vi "Login_Process.vi"(8 "error in (no error)":errorcluster, 11 "TopLevel in":refnum<class "TopLevel.lvclass">) -> (0 "error out":errorcluster, 3 "TopLevel out":refnum<class "TopLevel.lvclass">)   [LabVIEW 2022 SP3, in "TopLevel.lvclass"]
uses:
  TopLevel.lvclass
  Typedefs/UserLevel_withoutNone--Enum.ctl
  Typedefs/UserLevel--Enum.ctl
panel:
  out "Status":string
  in  "UserLevel":T1
  in  "LogIN":bool
  in  "Cancel":bool
  in  "Password":string
  in  "OK":bool
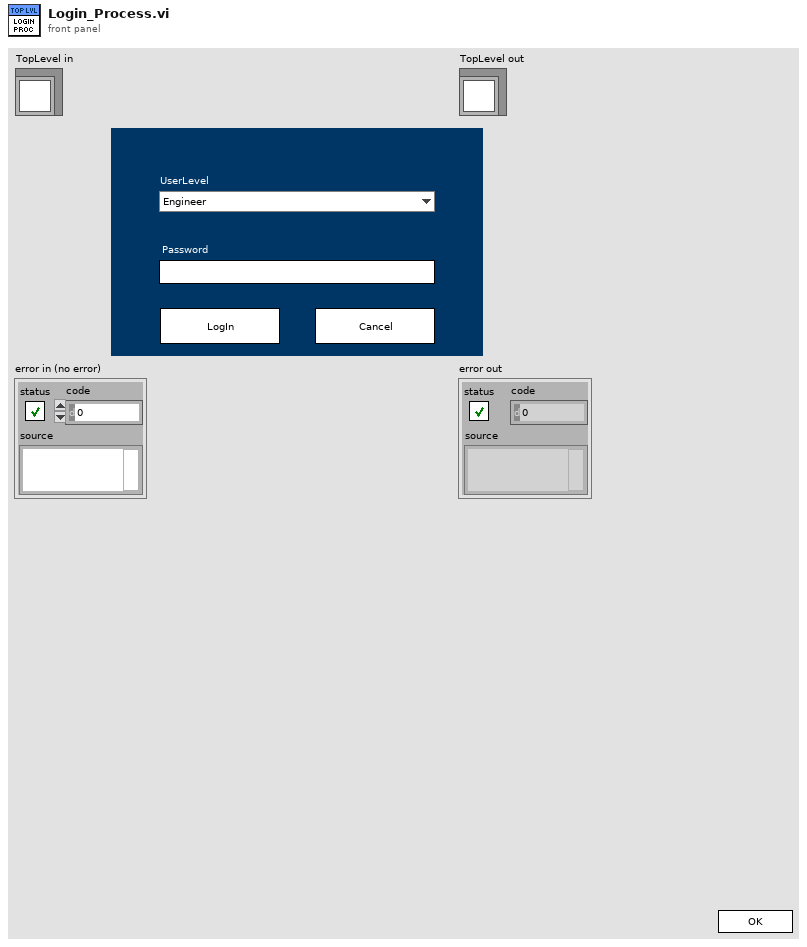
[diagram p1: front panel]
types:
  T1 = typedef "UserLevel_withoutNone--Enum.ctl" = enum16{"Engineer"}
  T2 = typedef "UserLevel--Enum.ctl" = enum16{"None", "Operator", "Engineer"}
  T3 = enum32{"Invalid", "Standard", "Closed", "Hidden", "Minimized", "Maximized"}
  T4 = enum32{"invalid app kind", "Development System", "Run Time System", "Student Edition", "Embedded LabVIEW", "Evaluation", "Custom"}
  T5 = cluster{"Core":cluster{"Current VI Reference":refnum<vi>, "Close Panel on Exit?":bool}, "TopLevel in":refnum<class "TopLevel.lvclass">, "Your string data":string}
  T6 = cluster{"Current VI Reference":refnum<vi>, "Close Panel on Exit?":bool}
  T7 = typedef "TopLevel.lvclass/UserEvents.ctl" = cluster{"API Incoming Event":refnum<user-event>, "API Executed Event":refnum<user-event>, "API Return Event":refnum<user-event>, "Exit Event":refnum<user-event>, "StatusChanged":refnum<user-event>, "DLP GUI Config Changed":refnum<user-event>, "AppEvent":refnum<user-event>, "Login Event":refnum<user-event>, "HeadPrimeStatusEvent":refnum<user-event>}
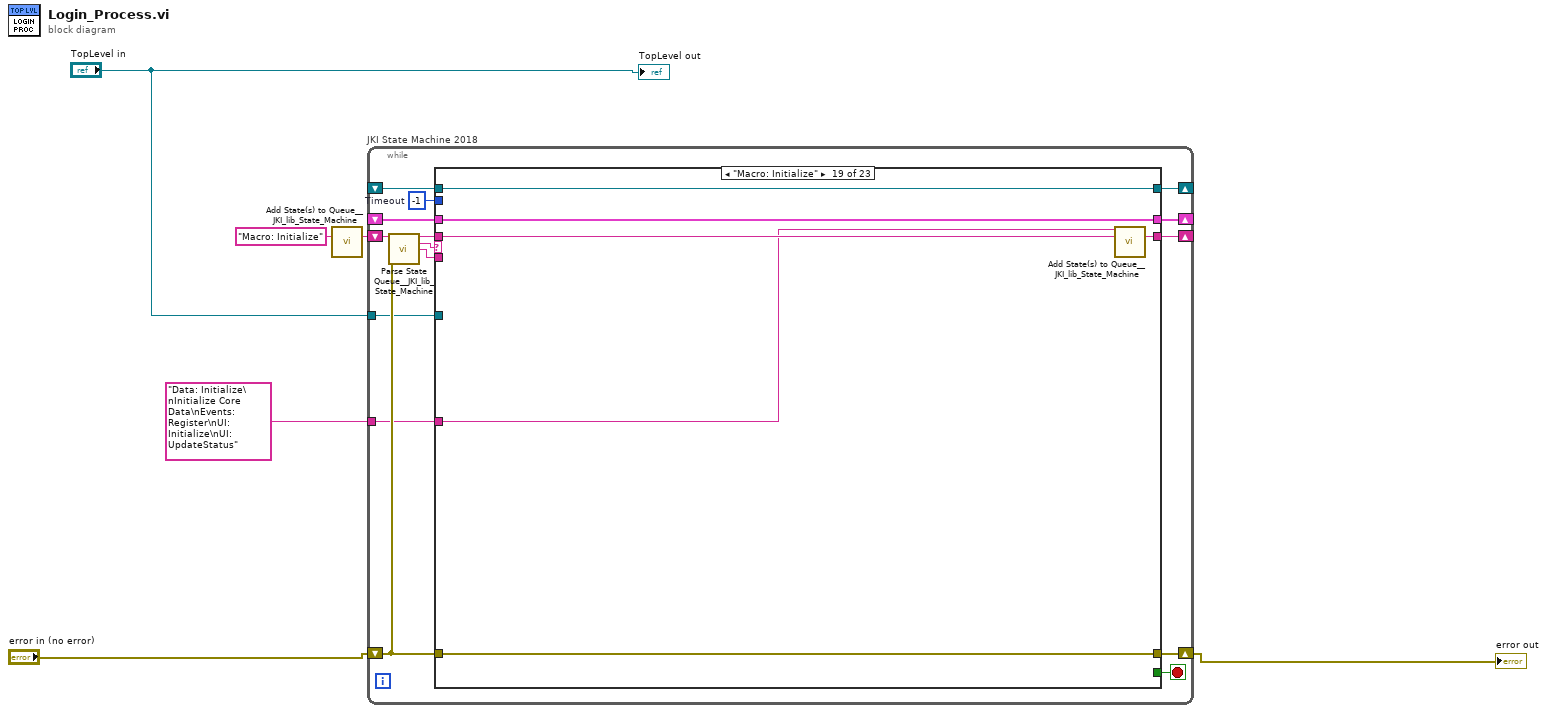
[diagram p0: block diagram]
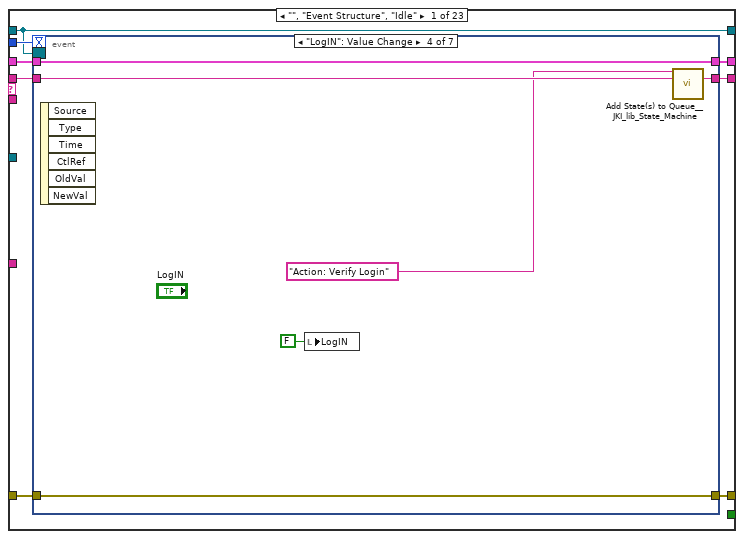
[diagram p2: hidden frame]
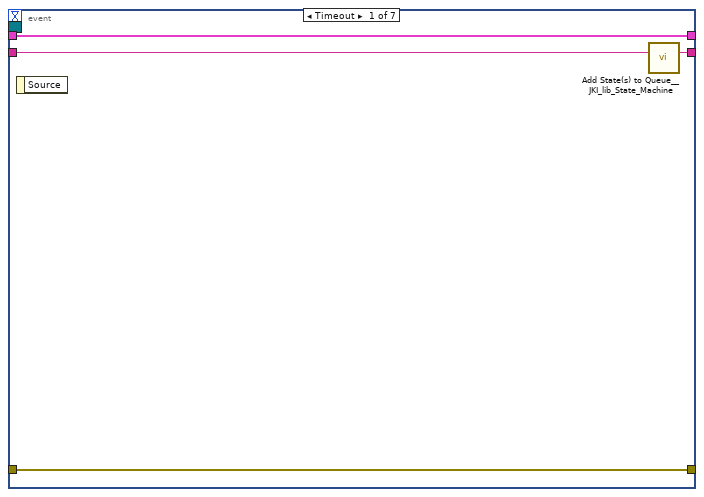
[diagram p3: hidden frame]
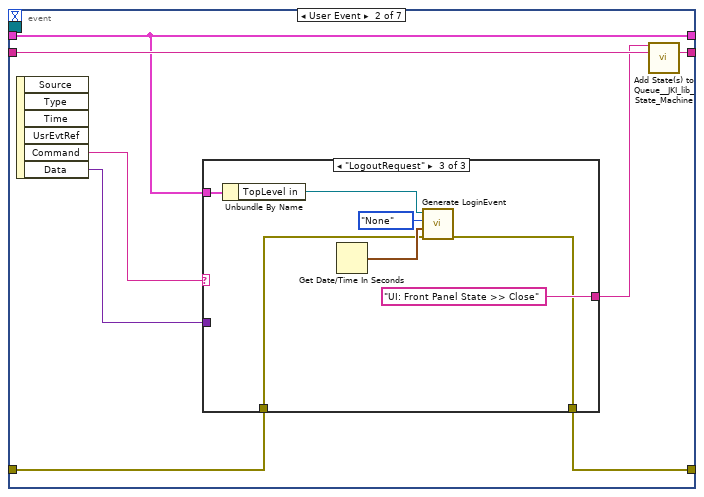
[diagram p4: hidden frame]
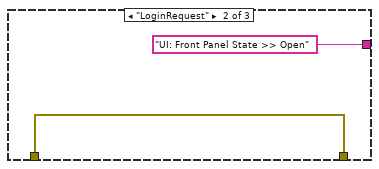
[diagram p6: hidden frame]
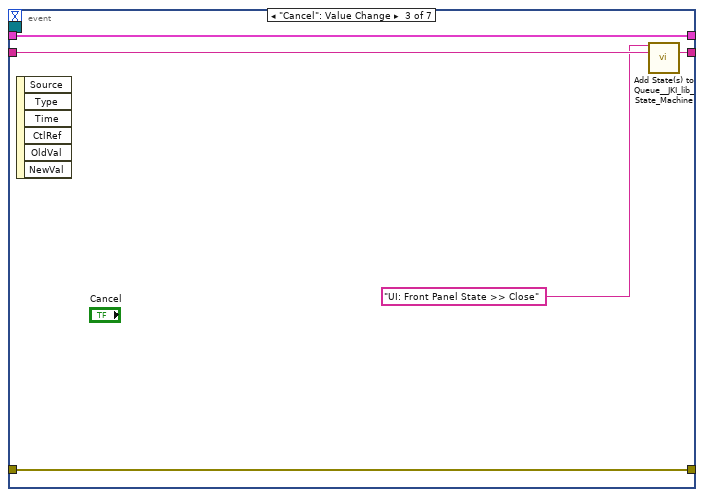
[diagram p7: hidden frame]
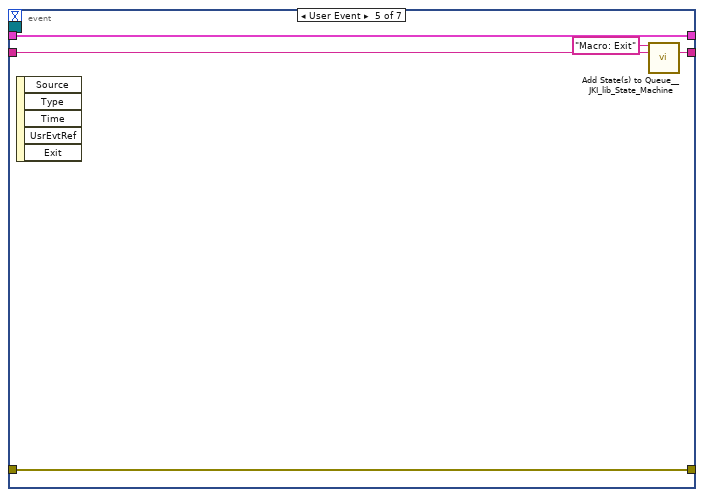
[diagram p8: hidden frame]
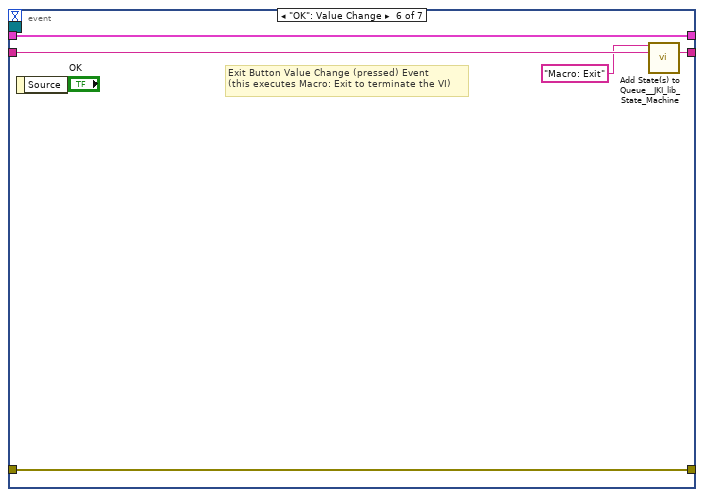
[diagram p9: hidden frame]
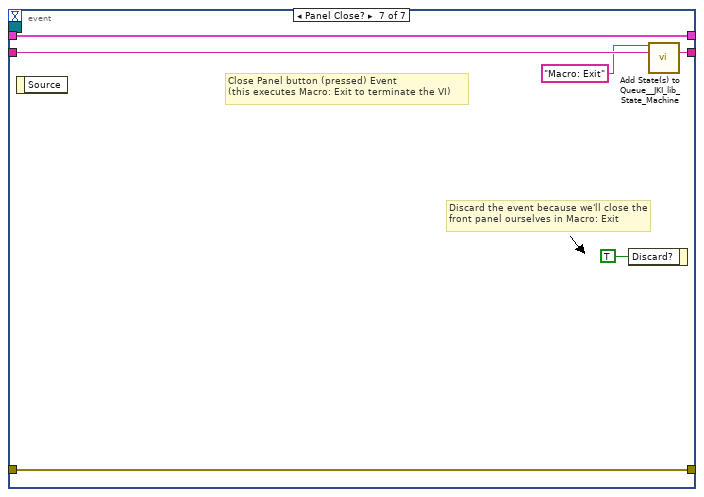
[diagram p10: hidden frame]
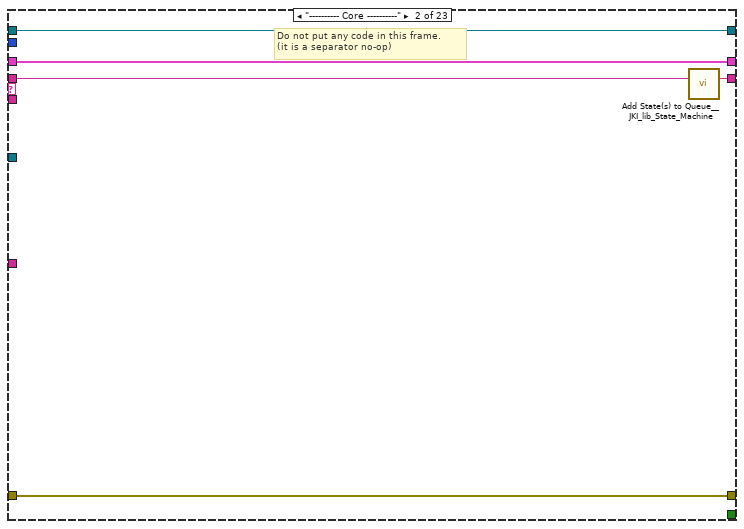
[diagram p11: hidden frame]
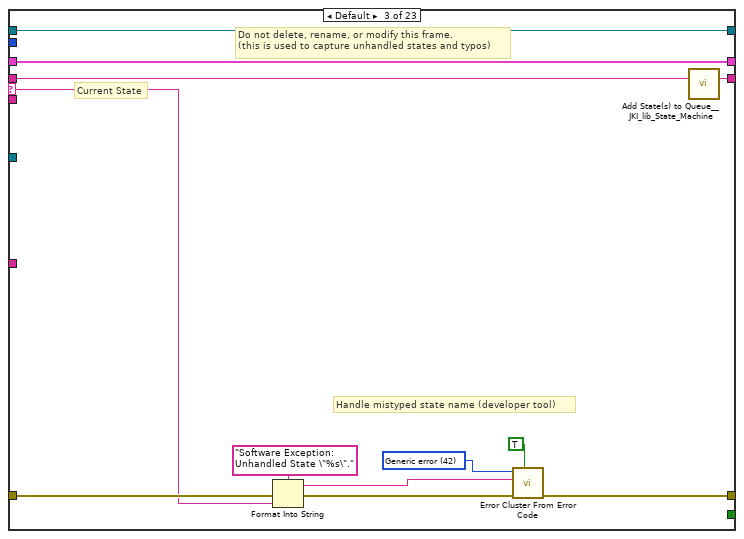
[diagram p12: hidden frame]
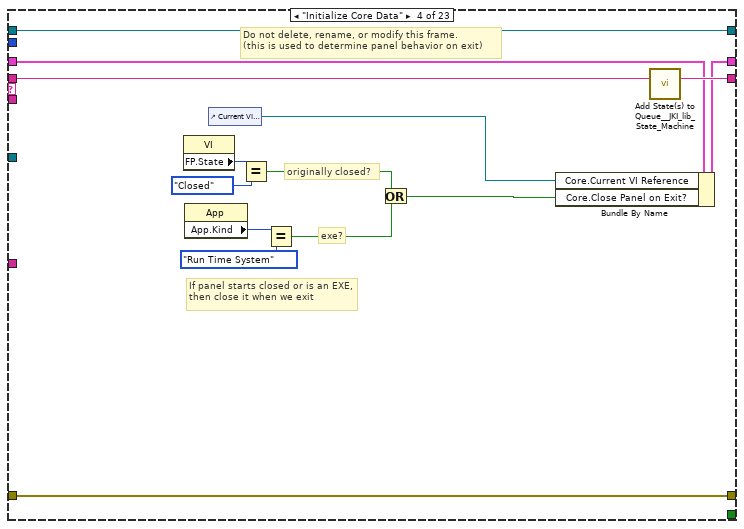
[diagram p13: hidden frame]
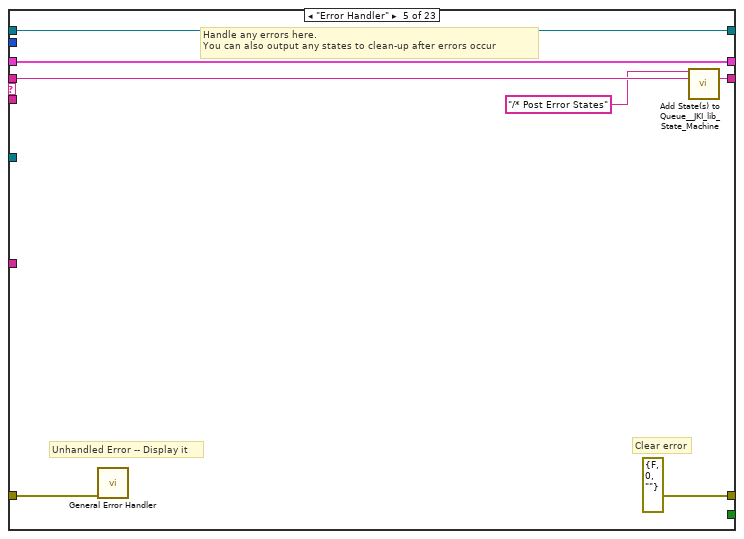
[diagram p14: hidden frame]
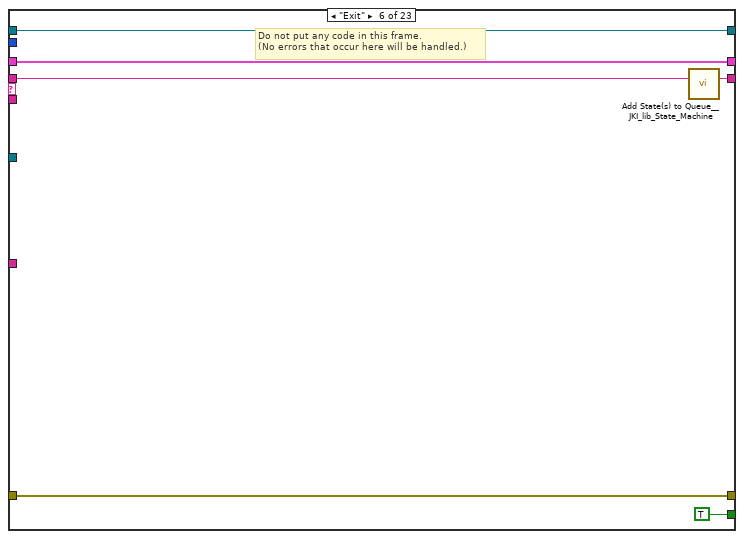
[diagram p15: hidden frame]
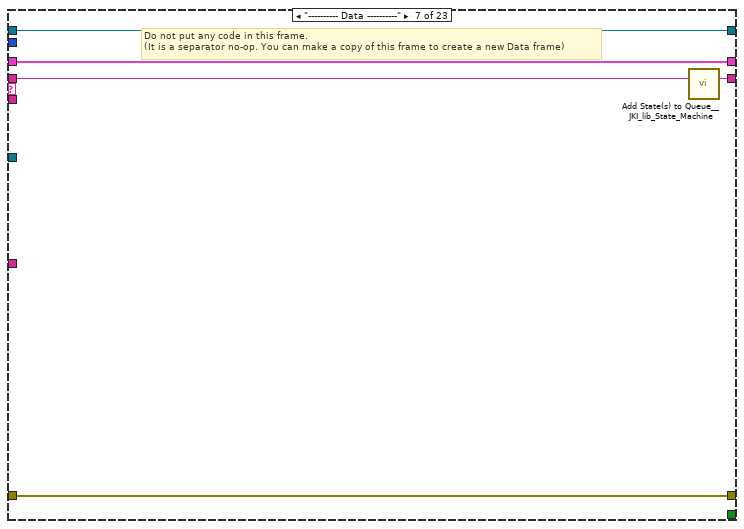
[diagram p16: hidden frame]
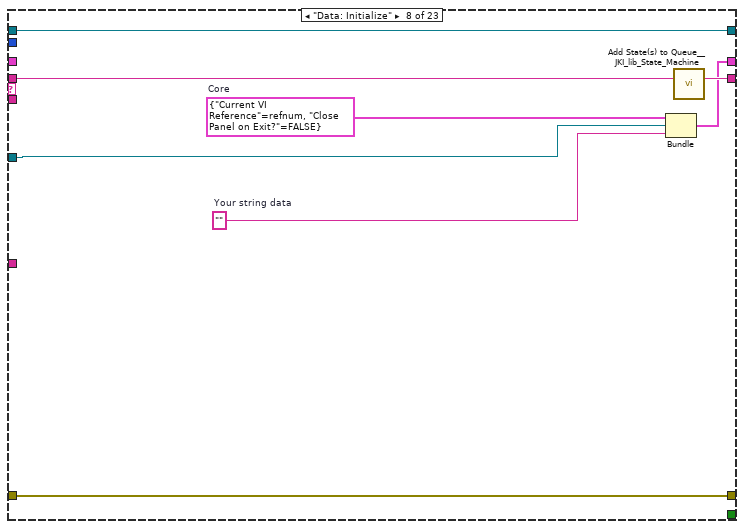
[diagram p17: hidden frame]
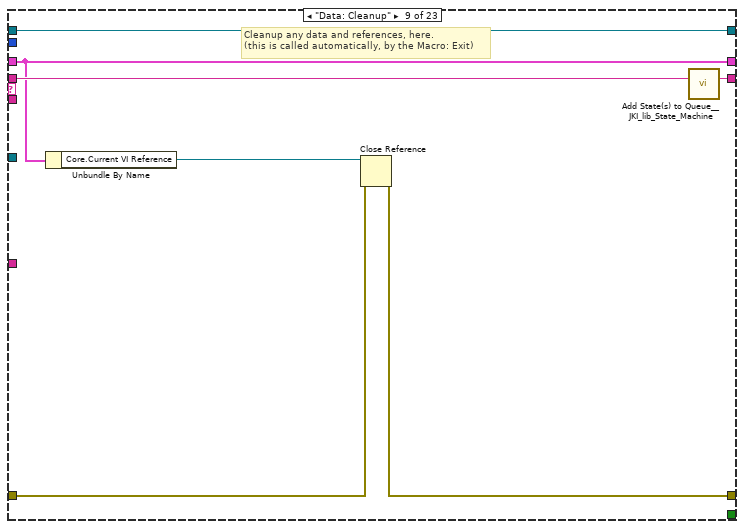
[diagram p18: hidden frame]
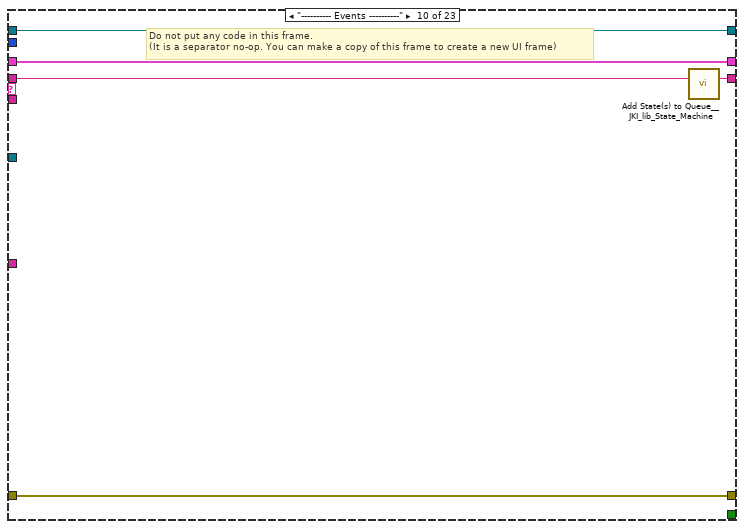
[diagram p19: hidden frame]
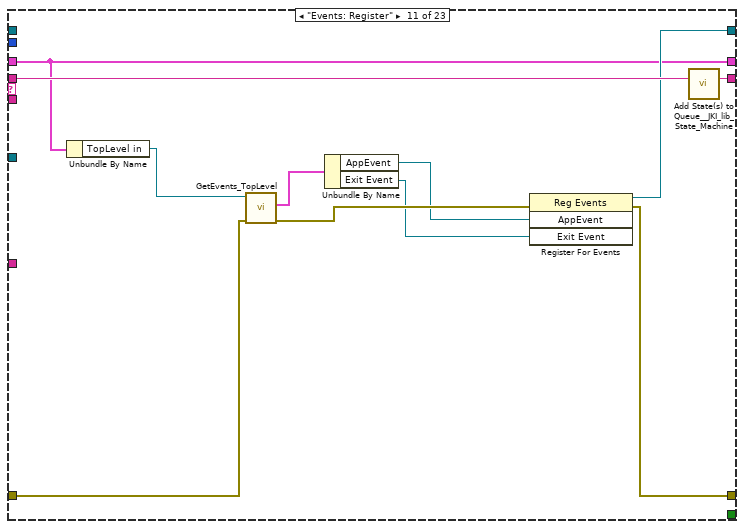
[diagram p20: hidden frame]
diagram:
  n1 = call <vilib>:"Add State(s) to Queue__JKI_lib_State_Machine.vi"("State(s) in (\"\")"="Macro: Initialize") -> ("States Out"=w6:string)  [unwired: 14 in]
  n2 = while "JKI State Machine 2018" {
    shift-right: [w14] -> _
    shift-left: _ -> [w13]
    shift-right: [w17] -> w3
    shift-left: "error in (no error)" -> [w11]
    shift-right: [w16] -> _
    shift-left: w6 -> [w18]
    tunnel: "TopLevel in" -> [w10]
    shift-right: [w9] -> _
    shift-left: _ -> [w8]
    tunnel: "Data: Initialize\nInitialize Core Data\nEvents: Register\nUI: Initialize\nUI: UpdateStatus" -> [w7]
    stop <- w15 stop-if-true
    w12 = -1  # Timeout
    n3 = call <vilib>:"Parse State Queue__JKI_lib_State_Machine.vi"("State Queue"=w18, "Error In (no error)"=w11) -> ("Remaining States"=w20:string, "Current State"=w21:string, "Arguments"=w19:string)  [unwired: 11 in]
    n4 = case shown="\"Macro: Initialize\"" w21 {
      selector: w21 -> [_ _ w85 _ _ _ _ _ _ _ _ _ _ _ _ _ _ _ _ _ _ _ _]
      tunnel: w20 -> [w29 w83 w89 w109 w116 w122 w127 w135 w142 w147 w158 w164 w169 w177 w187 w194 w206 w276 w282 w293 w298 w303 w315]
      tunnel: w19 -> [_ _ _ _ _ _ _ _ _ _ _ _ _ w171 _ w189 w200 _ _ _ _ _ _]
      tunnel: w13 -> [w27 w80 w87 w102 w113 w120 w124 _ w137 w144 w152 w162 w166 w174 w185 w192 w202 w273 w279 w290 w295 w300 w309]
      tunnel: [w26 w81 w91 w106 errorcluster {"status"=FALSE, "code"=0, "source"=""} ("error out") w119 w125 w132 w138 w145 w155 w159 w167 w175 w183 w190 w203 w274 w280 w291 w296 w301 w307] -> w17
      tunnel: w11 -> [w25 w81 w90 w106 w112 w119 w125 w132 w139 w145 w151 w160 w167 w175 w182 w191 w204 w274 w280 w291 w296 w301 w306]
      tunnel: [w28 w82 w88 w108 w115 w121 w126 w134 w141 w146 w157 w163 w168 w176 w186 w193 w205 w275 w281 w292 w297 w302 w314] -> w16
      tunnel: [_ _ _ _ _ TRUE _ _ _ _ _ _ _ _ _ _ _ _ _ _ _ _ _] -> w15
      tunnel: [w24 w80 w87 w107 w113 w120 w124 w133 w137 w144 w152 w162 w166 w174 w185 w192 w202 w273 w279 w290 w295 w300 w309] -> w14
      tunnel: w12 -> [w23 _ _ _ _ _ _ _ _ _ _ _ _ _ _ _ _ _ _ _ _ _ _]
      tunnel: w10 -> [_ _ _ _ _ _ _ w129 _ _ _ _ _ _ _ _ _ _ _ _ _ _ _]
      tunnel: [w22 w79 w84 w96 w110 w117 w123 w128 w136 w143 w156 w161 w165 w173 w184 w188 w199 w272 w278 w283 w294 w299 w313] -> w9
      tunnel: w8 -> [w22 w79 w84 w96 w110 w117 w123 w128 w136 w143 _ w161 w165 w173 w184 w188 w199 w272 w278 w283 w294 w299 w313]
      tunnel: w7 -> [_ _ _ _ _ _ _ _ _ _ _ _ _ _ _ _ _ _ w277 _ _ _ _]
      frame "", "Event Structure", "Idle" {
        n5 = event shown="[3] \"LogIN\": Value Change" {
          selector: w22 -> [_ _ _ _ _ _ _]
          dyn-events: _ -> [_ _ _ _ _ _ _]
          timeout: w23 -> [_ _ _ _ _ _ _]
          tunnel: w29 -> [w33 w41 w56 w62 w67 w72 w78]
          tunnel: [w32 w40 w55 w61 w66 w71 w77] -> w28
          tunnel: w27 -> [w30 w34 w53 w59 w64 w69 w75]
          tunnel: [w31 w36 w54 w60 w65 w70 w76] -> w26
          tunnel: w25 -> [w31 w35 w54 w60 w65 w70 w76]
          tunnel: [w30 w34 w53 w59 w64 w69 w75] -> w24
          event Timeout {
            n6 = event-data() -> ()  [unwired: 1 in, 1 out]
            n7 = call <vilib>:"Add State(s) to Queue__JKI_lib_State_Machine.vi"("State(s) in (\"\")"=w33) -> ("States Out"=w32:string)  [unwired: 14 in]
          }
          event User Event {
            n8 = event-data() -> ("Command"=w39:string, "Data"=w38:variant)  [unwired: 1 in, 4 out]
            n9 = case shown="\"LogoutRequest\"" w39 {
              tunnel: w38 -> [_ _ _]
              tunnel: [_ "UI: Front Panel State >> Open" "UI: Front Panel State >> Close"] -> w37
              tunnel: w35 -> [w42 w43 w48]
              tunnel: [w42 w43 w47] -> w36
              tunnel: w34 -> [_ _ w46]
              frame Default {
              }
              frame "LoginRequest" {
              }
              frame "LogoutRequest" {
                n10 = Unbundle By Name(w46) -> ("TopLevel in"=w45:refnum<class "TopLevel.lvclass">)
                n11 = Get Date/Time In Seconds() -> (seconds since 1Jan1904=w49:timestamp)
                n12 = call-dynamic "Generate LoginEvent.vi"("error in (no error)"=w48, "Login Time"=w49, "UserLevel"=UserLevel--Enum."None", "TopLevel in"=w45) -> ("error out"=w47:errorcluster)  [unwired: 6 in, 1 out]
              }
            }
            n13 = call <vilib>:"Add State(s) to Queue__JKI_lib_State_Machine.vi"("State(s) in Front (\"\")"=w37, "State(s) in (\"\")"=w41) -> ("States Out"=w40:string)  [unwired: 13 in]
          }
          event "Cancel": Value Change {
            n14 = event-data() -> ()  [unwired: 1 in, 6 out]
            n15 = call <vilib>:"Add State(s) to Queue__JKI_lib_State_Machine.vi"("State(s) in Front (\"\")"="UI: Front Panel State >> Close", "State(s) in (\"\")"=w56) -> ("States Out"=w55:string)  [unwired: 13 in]
          }
          event "LogIN": Value Change {
            n16 = event-data() -> ()  [unwired: 1 in, 6 out]
            n17 = local write "LogIN"(FALSE ("LogIN")) -> ()
            n18 = call <vilib>:"Add State(s) to Queue__JKI_lib_State_Machine.vi"("State(s) in Front (\"\")"="Action: Verify Login" ("State(s) in Front (\"\")"), "State(s) in (\"\")"=w62) -> ("States Out"=w61:string)  [unwired: 13 in]
          }
          event User Event {
            n19 = event-data() -> ()  [unwired: 1 in, 5 out]
            n20 = call <vilib>:"Add State(s) to Queue__JKI_lib_State_Machine.vi"("State(s) in Front (\"\")"="Macro: Exit" ("State(s) in Front (\"\")"), "State(s) in (\"\")"=w67) -> ("States Out"=w66:string)  [unwired: 13 in]
          }
          event "OK": Value Change {
            # "Exit Button Value Change (pressed) Event\n(this executes Macro: Exit to terminate the VI)"
            n21 = event-data() -> ()  [unwired: 1 in, 1 out]
            n22 = call <vilib>:"Add State(s) to Queue__JKI_lib_State_Machine.vi"("State(s) in Front (\"\")"="Macro: Exit", "State(s) in (\"\")"=w72) -> ("States Out"=w71:string)  [unwired: 13 in]
          }
          event Panel Close? {
            # "Discard the event because we'll close the front panel ourselves in Macro: Exit"
            # "Close Panel button (pressed) Event\n(this executes Macro: Exit to terminate the VI)"
            n23 = event-data() -> ()  [unwired: 1 in, 1 out]
            n24 = event-data("Discard?"=TRUE) -> ()  [unwired: 1 in, 1 out]
            n25 = call <vilib>:"Add State(s) to Queue__JKI_lib_State_Machine.vi"("State(s) in Front (\"\")"="Macro: Exit", "State(s) in (\"\")"=w78) -> ("States Out"=w77:string)  [unwired: 13 in]
          }
        }
      }
      frame "---------- Core ----------" {
        # "Do not put any code in this frame.\n(it is a separator no-op)"
        n26 = call <vilib>:"Add State(s) to Queue__JKI_lib_State_Machine.vi"("State(s) in (\"\")"=w83) -> ("States Out"=w82:string)  [unwired: 14 in]
      }
      frame Default {
        w94 = 42 items=["No error", "Argument error", "Memory is full", "Out of zone", "End of file", "File already open", "Generic file I/O error", "File not found", "File permission error", "Disk is full", "Duplicate path", "Too many files open", "System feature not enabled", "Resource file not found", "Cannot add resource", "Resource not found", "Image not found", "Image memory error", "Pen does not exist", "Config type invalid", "Config token not found", "Config parse error", "Config memory error", "Bad external code format", "Bad external code offset", "External code not present", "Null window", "Destroy window error", "Null menu", "Print aborted", "Bad print record", "Print driver error", "Windows error during printing", "Memory error during printing", "Print dialog error", "Generic print error", "Invalid device refnum", "Device not found", "Device parameter error", "Device unit error", "Cannot open device", "Device call aborted", "Generic error", "Cancelled by user", "Object ID too low", "Object ID too high", "Object not in heap", "Unknown heap", "Unknown object (invalid DefProc)", "Unknown object (DefProc not in table)", "Message out of range", "Invalid (null) method", "Unknown message", "Manager call not supported", "Bad address", "Network operation in progress", "Network operation timed out", "Connection is busy", "Network attribute not supported", "Network error", "Address in use", "System out of memory", "Connection aborted", "Connection refused", "Not connected", "Already connected", "Connection closed", "Initialization error (interapplication manager)", "Bad occurrence", "Wait on unbound occurrence handler", "Occurrence queue overflow", "Datalog type conflict", "Unused", "Unrecognized type (interapplication manager)", "Memory corrupt", "Failed to make temporary DLL", "Old CIN version", "Drag socket not found", "Failed to load drop-object", "Failed to register OLE object", "Failed to release OLE object", "Format specifier type mismatch", "Unknown format specifier", "Too few format specifiers", "Too many format specifiers", "Scan failed", "Newer CIN version", "Error converting to variant", "Runtime menu error", "Password tampered", "Variant attribute not found", "Incompatible variant data type", "Event data is not available", "Event Store is not present", "Occurrence is not found", "Event Queue is not created", "Event info is not available", "Refnum passed is NULL", "Error retrieving Class GUID", "Error retrieving CoClass GUID", "Error retrieving TypeLib GUID.", "Bad built application magic bytes.", "Specific driver is different from the specific driver associated with the Logical Name.", "There is no session opened to the class driver.", "Max Error", "MAX - Error with config objects", "MAX - Error loading configuration", "MAX - Group not supported"]
        # "Current State"
        # "Do not delete, rename, or modify this frame.\n(this is used to capture unhandled states and typos)"
        # "Handle mistyped state name (developer tool)"
        n27 = Format Into String(format string="Software Exception: Unhandled State \"%s\"." ("message"), error in=w90, w85) -> (resulting string=w93:string, error out=w92:errorcluster)  [unwired: 1 in]
        n28 = call <vilib>:"Error Cluster From Error Code.vi"("show call chain? (False)"=TRUE, "error in (no error)"=w92, "error message (\"\")"=w93, "error code (0)"=w94) -> ("error out"=w91:errorcluster)  [unwired: 5 in]
        n29 = call <vilib>:"Add State(s) to Queue__JKI_lib_State_Machine.vi"("State(s) in (\"\")"=w89) -> ("States Out"=w88:string)  [unwired: 14 in]
      }
      frame "Initialize Core Data" {
        # "Do not delete, rename, or modify this frame.\n(this is used to determine panel behavior on exit)"
        # "originally closed?"
        # "exe?"
        # "If panel starts closed or is an EXE, then close it when we exit"
        n30 = property class="VI"() -> ("FP.State"=w99:T3)  [unwired: 2 in, 2 out]
        n31 = property class="App"() -> ("App.Kind"=w105:T4)  [unwired: 2 in, 2 out]
        n32 = control-ref of="Current VI Reference"() -> (w100:refnum<vi>)
        n33 = Equal?(x=w99, y=T3."Closed" ("Front Panel Window:State")) -> (x = y?=w97:bool)
        n34 = Equal?(x=w105, y=T4."Run Time System" ("Application:Kind")) -> (x = y?=w103:bool)
        n35 = Or(x=w97, y=w103) -> (x .or. y?=w101:bool)
        n36 = Bundle By Name(cluster=w102, "Core.Current VI Reference"=w100, "Core.Close Panel on Exit?"=w101) -> (w107:T5)
        n37 = call <vilib>:"Add State(s) to Queue__JKI_lib_State_Machine.vi"("State(s) in (\"\")"=w109) -> ("States Out"=w108:string)  [unwired: 14 in]
      }
      frame "Error Handler" {
        # "Unhandled Error -- Display it"
        # "Handle any errors here.\nYou can also output any states to clean-up after errors occur"
        # "Clear error"
        n38 = call <vilib>:"General Error Handler.vi"("error in (no error)"=w112) -> ()  [unwired: 10 in, 5 out]
        n39 = call <vilib>:"Add State(s) to Queue__JKI_lib_State_Machine.vi"("State(s) in Front (\"\")"="/* Post Error States", "State(s) in (\"\")"=w116) -> ("States Out"=w115:string)  [unwired: 13 in]
      }
      frame "Exit" {
        # "Do not put any code in this frame.\n(No errors that occur here will be handled.)"
        n40 = call <vilib>:"Add State(s) to Queue__JKI_lib_State_Machine.vi"("State(s) in (\"\")"=w122) -> ("States Out"=w121:string)  [unwired: 14 in]
      }
      frame "---------- Data ----------" {
        # "Do not put any code in this frame.\n(It is a separator no-op. You can make a copy of this frame to create a new Data frame)"
        n41 = call <vilib>:"Add State(s) to Queue__JKI_lib_State_Machine.vi"("State(s) in (\"\")"=w127) -> ("States Out"=w126:string)  [unwired: 14 in]
      }
      frame "Data: Initialize" {
        w130 = T6 {"Current VI Reference"=refnum, "Close Panel on Exit?"=FALSE}  # Core
        w131 = ""  # Your string data
        n42 = Bundle("Core"=w130, "TopLevel in"=w129, "Your string data"=w131) -> (w133:T5)  [unwired: 1 in]
        n43 = call <vilib>:"Add State(s) to Queue__JKI_lib_State_Machine.vi"("State(s) in (\"\")"=w135) -> ("States Out"=w134:string)  [unwired: 14 in]
      }
      frame "Data: Cleanup" {
        # "Cleanup any data and references, here.\n(this is called automatically, by the Macro: Exit)"
        n44 = Unbundle By Name(w137) -> ("Core.Current VI Reference"=w140:refnum<vi>)
        n45 = Close Reference(reference=w140, error in (no error)=w139) -> (error out=w138:errorcluster)
        n46 = call <vilib>:"Add State(s) to Queue__JKI_lib_State_Machine.vi"("State(s) in (\"\")"=w142) -> ("States Out"=w141:string)  [unwired: 14 in]
      }
      frame "---------- Events ----------" {
        # "Do not put any code in this frame.\n(It is a separator no-op. You can make a copy of this frame to create a new UI frame)"
        n47 = call <vilib>:"Add State(s) to Queue__JKI_lib_State_Machine.vi"("State(s) in (\"\")"=w147) -> ("States Out"=w146:string)  [unwired: 14 in]
      }
      frame "Events: Register" {
        n48 = Unbundle By Name(w152) -> ("TopLevel in"=w153:refnum<class "TopLevel.lvclass">)
        n49 = call-dynamic "GetEvents_TopLevel.vi"("error in (no error)"=w151, "TopLevel in"=w153) -> ("error out"=w150:errorcluster, "UserEvents"=w154:T7)  [unwired: 7 in, 1 out]
        n50 = Unbundle By Name(w154) -> ("AppEvent"=w149:refnum<user-event>, "Exit Event"=w148:refnum<user-event>)
        n51 = register-events(error in=w150, w149, w148) -> (reference out=w156:refnum<event-registration>, error out=w155:errorcluster)  [unwired: 1 in]
        n52 = call <vilib>:"Add State(s) to Queue__JKI_lib_State_Machine.vi"("State(s) in (\"\")"=w158) -> ("States Out"=w157:string)  [unwired: 14 in]
      }
      frame "Events: Unregister" {
        # "Do not put any code in this frame.\n(It is a separator no-op. You can make a copy of this frame to create a new UI frame)"
        n53 = Unregister For Events(event registration refnum=w161, error in=w160) -> (error out=w159:errorcluster)
        n54 = call <vilib>:"Add State(s) to Queue__JKI_lib_State_Machine.vi"("State(s) in (\"\")"=w164) -> ("States Out"=w163:string)  [unwired: 14 in]
      }
      frame "---------- UI ----------" {
        # "Do not put any code in this frame.\n(It is a separator no-op. You can make a copy of this frame to create a new UI frame)"
        n55 = call <vilib>:"Add State(s) to Queue__JKI_lib_State_Machine.vi"("State(s) in (\"\")"=w169) -> ("States Out"=w168:string)  [unwired: 14 in]
      }
      frame "UI: UpdateStatus" {
        # "Do not put any code in this frame.\n(It is a separator no-op. You can make a copy of this frame to create a new UI frame)"
        n56 = Empty String/Path?(string/path=w171) -> (empty?=w172:bool)
        n57 = case shown="True" w172 {
          tunnel: w171 -> [w179 _]
          tunnel: [TRUE ("Visible") FALSE ("Visible")] -> w170
          frame False {
            "Status" <- w179
          }
          frame True {
            n58 = local write "Status"("" ("Status")) -> ()
          }
        }
        n59 = property on="Status" class="Str"("Visible"=w170) -> ()  [unwired: 2 in, 2 out]
        n60 = call <vilib>:"Add State(s) to Queue__JKI_lib_State_Machine.vi"("State(s) in (\"\")"=w177) -> ("States Out"=w176:string)  [unwired: 14 in]
      }
      frame "UI: Initialize" {
        n61 = call <userlib>:"Fit VI window to Largest Dec__ogtk.vi"("error in (no error)"=w182) -> ("error out"=w183:errorcluster)  [unwired: 5 in, 1 out]
        n62 = call <vilib>:"Add State(s) to Queue__JKI_lib_State_Machine.vi"("State(s) in (\"\")"=w187) -> ("States Out"=w186:string)  [unwired: 14 in]
      }
      frame "UI: Cursor Set" {
        # "Argument"
        # "Set and Unset Cursor Busy.\n(Usage: \"UI: Cursor Set >> Busy|Idle\")"
        n63 = case shown="\"Idle\", Default" w189 {
          tunnel: w191 -> [w196 w198]
          tunnel: [w195 w197] -> w190
          frame "Idle", Default {
            n64 = call <vilib>:"Unset Busy.vi"("error in (no error)"=w196) -> ("error out"=w195:errorcluster)  [unwired: 10 in]
          }
          frame "Busy" {
            n65 = call <vilib>:"Set Busy.vi"("error in (no error)"=w198) -> ("error out"=w197:errorcluster)  [unwired: 9 in, 1 out]
          }
        }
        n66 = call <vilib>:"Add State(s) to Queue__JKI_lib_State_Machine.vi"("State(s) in (\"\")"=w194) -> ("States Out"=w193:string)  [unwired: 14 in]
      }
      frame "UI: Front Panel State" {
        # "Argument"
        # "Set Front Panel Open or Closed\n(Usage: \"UI: Front Panel State >> Open|Close\")"
        n67 = Unbundle By Name(w202) -> ("Core.Current VI Reference"=w201:refnum<vi>)
        n68 = case shown="\"Minimize\", \"Minimized\"" w200 {
          tunnel: w204 -> [w212 w227 w238 w251 w264]
          tunnel: [w214 w228 w240 w253 w266] -> w203
          tunnel: w201 -> [w213 w225 w239 w252 w265]
          frame "Open", "Standard", Default {
            w207 = T3."Standard" ("State")
            n69 = property class="VI"(reference=w213, error in=w212) -> (reference out=w210:refnum<vi>, error out=w211:errorcluster, "FP.State"=w209:T3)
            n70 = Not Equal?(x=w209, y=w207) -> (x != y?=w208:bool)
            n71 = case shown="True" w208 {
              tunnel: [w218 w220] -> w214
              tunnel: w211 -> [w217 w220]
              tunnel: w210 -> [w216 _]
              tunnel: w207 -> [w215 _]
              frame True {
                n72 = invoke class="VI" method="FP.Open"(reference=w216, error in=w217, "Activate"=TRUE, "State"=w215) -> (error out=w218:errorcluster)  [unwired: 1 in, 4 out]
              }
              frame False {
              }
            }
          }
          frame "Close", "Closed" {
            n73 = property class="VI"(reference=w225, error in=w227) -> (reference out=w224:refnum<vi>, error out=w226:errorcluster, "FP.State"=w222:T3)
            n74 = Not Equal?(x=w222, y=T3."Closed" ("Front Panel Window:State")) -> (x != y?=w221:bool)
            n75 = case shown="True" w221 {
              tunnel: [w229 w232] -> w228
              tunnel: w226 -> [w229 w231]
              tunnel: w224 -> [_ w230]
              frame False {
              }
              frame True {
                n76 = invoke class="VI" method="FP.Close"(reference=w230, error in=w231) -> (error out=w232:errorcluster)  [unwired: 1 in, 2 out]
              }
            }
          }
          frame "Hidden", "Hide" {
            w233 = T3."Hidden" ("State")
            n77 = property class="VI"(reference=w239, error in=w238) -> (reference out=w236:refnum<vi>, error out=w237:errorcluster, "FP.State"=w235:T3)
            n78 = Not Equal?(x=w235, y=w233) -> (x != y?=w234:bool)
            n79 = case shown="True" w234 {
              tunnel: [w244 w245] -> w240
              tunnel: w237 -> [w243 w245]
              tunnel: w236 -> [w242 _]
              tunnel: w233 -> [w241 _]
              frame True {
                n80 = invoke class="VI" method="FP.Open"(reference=w242, error in=w243, "State"=w241) -> (error out=w244:errorcluster)  [unwired: 2 in, 4 out]
              }
              frame False {
              }
            }
          }
          frame "Minimize", "Minimized" {
            w246 = T3."Minimized" ("State")
            n81 = property class="VI"(reference=w252, error in=w251) -> (reference out=w249:refnum<vi>, error out=w250:errorcluster, "FP.State"=w248:T3)
            n82 = Not Equal?(x=w248, y=w246) -> (x != y?=w247:bool)
            n83 = case shown="True" w247 {
              tunnel: [w257 w258] -> w253
              tunnel: w250 -> [w256 w258]
              tunnel: w249 -> [w255 _]
              tunnel: w246 -> [w254 _]
              frame True {
                n84 = invoke class="VI" method="FP.Open"(reference=w255, error in=w256, "State"=w254) -> (error out=w257:errorcluster)  [unwired: 2 in, 4 out]
              }
              frame False {
              }
            }
          }
          frame "Maximize", "Maximized" {
            w259 = T3."Maximized" ("State")
            n85 = property class="VI"(reference=w265, error in=w264) -> (reference out=w262:refnum<vi>, error out=w263:errorcluster, "FP.State"=w261:T3)
            n86 = Not Equal?(x=w261, y=w259) -> (x != y?=w260:bool)
            n87 = case shown="True" w260 {
              tunnel: [w270 w271] -> w266
              tunnel: w263 -> [w269 w271]
              tunnel: w262 -> [w268 _]
              tunnel: w259 -> [w267 _]
              frame True {
                n88 = invoke class="VI" method="FP.Open"(reference=w268, error in=w269, "State"=w267) -> (error out=w270:errorcluster)  [unwired: 2 in, 4 out]
              }
              frame False {
              }
            }
          }
        }
        n89 = call <vilib>:"Add State(s) to Queue__JKI_lib_State_Machine.vi"("State(s) in (\"\")"=w206) -> ("States Out"=w205:string)  [unwired: 14 in]
      }
      frame "---------- Macro ----------" {
        # "Do not put any code in this frame.\n(It is a separator no-op. You can make a copy of this frame to create a new Macro frame)"
        n90 = call <vilib>:"Add State(s) to Queue__JKI_lib_State_Machine.vi"("State(s) in (\"\")"=w276) -> ("States Out"=w275:string)  [unwired: 14 in]
      }
      frame "Macro: Initialize" {
        n91 = call <vilib>:"Add State(s) to Queue__JKI_lib_State_Machine.vi"("State(s) in Front (\"\")"=w277, "State(s) in (\"\")"=w282) -> ("States Out"=w281:string)  [unwired: 13 in]
      }
      frame "Macro: Exit" {
        # "Exit Macro\n(This is called once, when the VI exits)"
        n92 = Unbundle By Name(w290) -> ("Core.Close Panel on Exit?"=w289:bool)
        n93 = Select(t="UI: Front Panel State >> Close", s=w289, f="") -> (s? t:f=w286:string)
        n94 = call <vilib>:"Add State(s) to Queue__JKI_lib_State_Machine.vi"("State(s) in (\"\")"=w286, "State(s) at Back (\"\")"="Data: Cleanup\nEvents: Unregister\nExit") -> ("States Out"=w284:string)  [unwired: 13 in]
        n95 = call <vilib>:"Add State(s) to Queue__JKI_lib_State_Machine.vi"("State(s) in Front (\"\")"=w284, "State(s) in (\"\")"=w293) -> ("States Out"=w292:string)  [unwired: 13 in]
      }
      frame "----------Action----------" {
        # "Template Separator\n(You can make a copy of, or modify, this frame)"
        n96 = call <vilib>:"Add State(s) to Queue__JKI_lib_State_Machine.vi"("State(s) in (\"\")"=w298) -> ("States Out"=w297:string)  [unwired: 14 in]
      }
      frame "Process: Sync" {
        n97 = call <vilib>:"Add State(s) to Queue__JKI_lib_State_Machine.vi"("State(s) in (\"\")"=w303) -> ("States Out"=w302:string)  [unwired: 14 in]
      }
      frame "Action: Verify Login" {
        n98 = Unbundle By Name(w309) -> ("TopLevel in"=w308:refnum<class "TopLevel.lvclass">)
        n99 = case shown="\"Engineer\"" "UserLevel" {
          tunnel: "Password" -> [_ w329]
          tunnel: [TRUE w327] -> w310
          tunnel: [UserLevel--Enum."None" ("UserLevel") UserLevel--Enum."Engineer" ("UserLevel")] -> w305
          frame Default {
          }
          frame "Engineer" {
            n100 = Equal?(x=w329, y="Engr") -> (x = y?=w327:bool)
          }
        }
        n101 = case shown="False" w310 {
          tunnel: w308 -> [_ w322]
          tunnel: w306 -> [w317 w321]
          tunnel: [w317 w320] -> w307
          tunnel: w305 -> [_ w319]
          tunnel: ["UI: UpdateStatus>>Invalid Password" ("State(s) in Front (\"\")") "UI: Front Panel State >> Close" ("State(s) in Front (\"\")")] -> w304
          frame False {
            (unwired) "" ("message")
          }
          frame True {
            n102 = Get Date/Time In Seconds() -> (seconds since 1Jan1904=w323:timestamp)
            n103 = call-dynamic "Generate LoginEvent.vi"("error in (no error)"=w321, "Login Time"=w323, "UserLevel"=w319, "TopLevel in"=w322) -> ("error out"=w320:errorcluster)  [unwired: 6 in, 1 out]
          }
        }
        n104 = call <vilib>:"Add State(s) to Queue__JKI_lib_State_Machine.vi"("State(s) in Front (\"\")"=w304, "State(s) in (\"\")"=w315) -> ("States Out"=w314:string)  [unwired: 13 in]
      }
    }
  }
  "error out" <- w3
  "TopLevel out" <- "TopLevel in"
